vi "FillianVI.vi"() -> ()   [LabVIEW 2015]
uses:
  <vilib>/Utility/error.llb/Error Cluster From Error Code.vi
  <vilib>/ErrorRing/Error Ring.xnode
panel:
  out "Minimum voltage":dbl
  out "Max voltage":dbl
  out "Maximum temp":dbl
  out "Minimum temp":dbl
  out "Mean Temperature":dbl
  out "Mean voltage":dbl
  out "Warnings":errorcluster
  out "temp bat timeout":bool
  out "volt bat timeout":bool
  out "volt link timeout":bool
  out "temp link timeout":bool
  out "Link Quality 2":sgl
  out "Battery Voltage 2":sgl
  out "Battery Voltage":sgl
  out "Link Quality":sgl
  out "Voltage":sgl(graph)
  in  "stop":bool
  out "Temperature":sgl(graph)
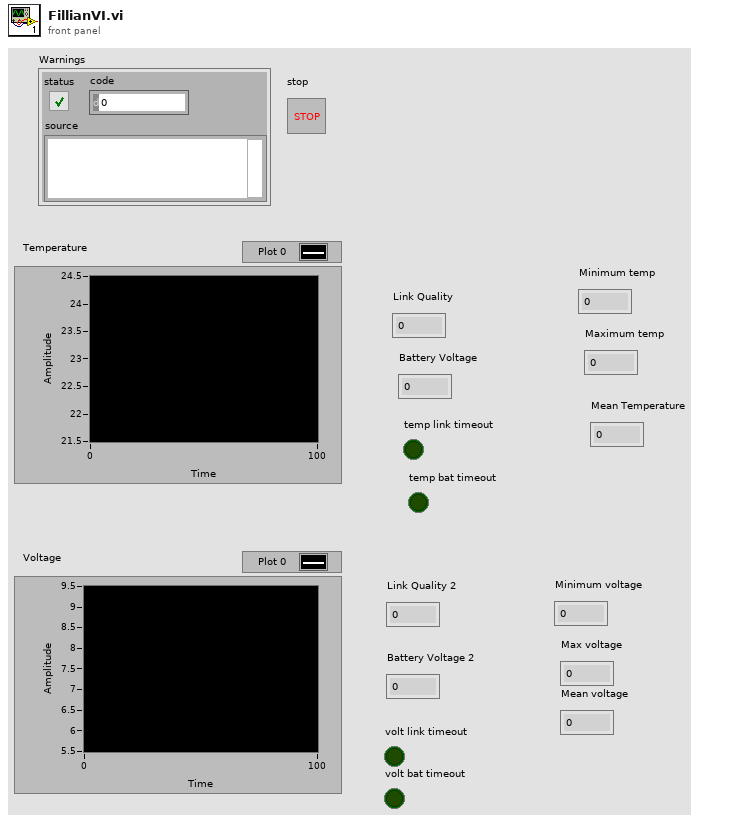
[diagram p1: front panel]
types:
  T1 = enum16{"open", "replace", "create", "open or create", "replace or create", "replace or create with confirmation"}
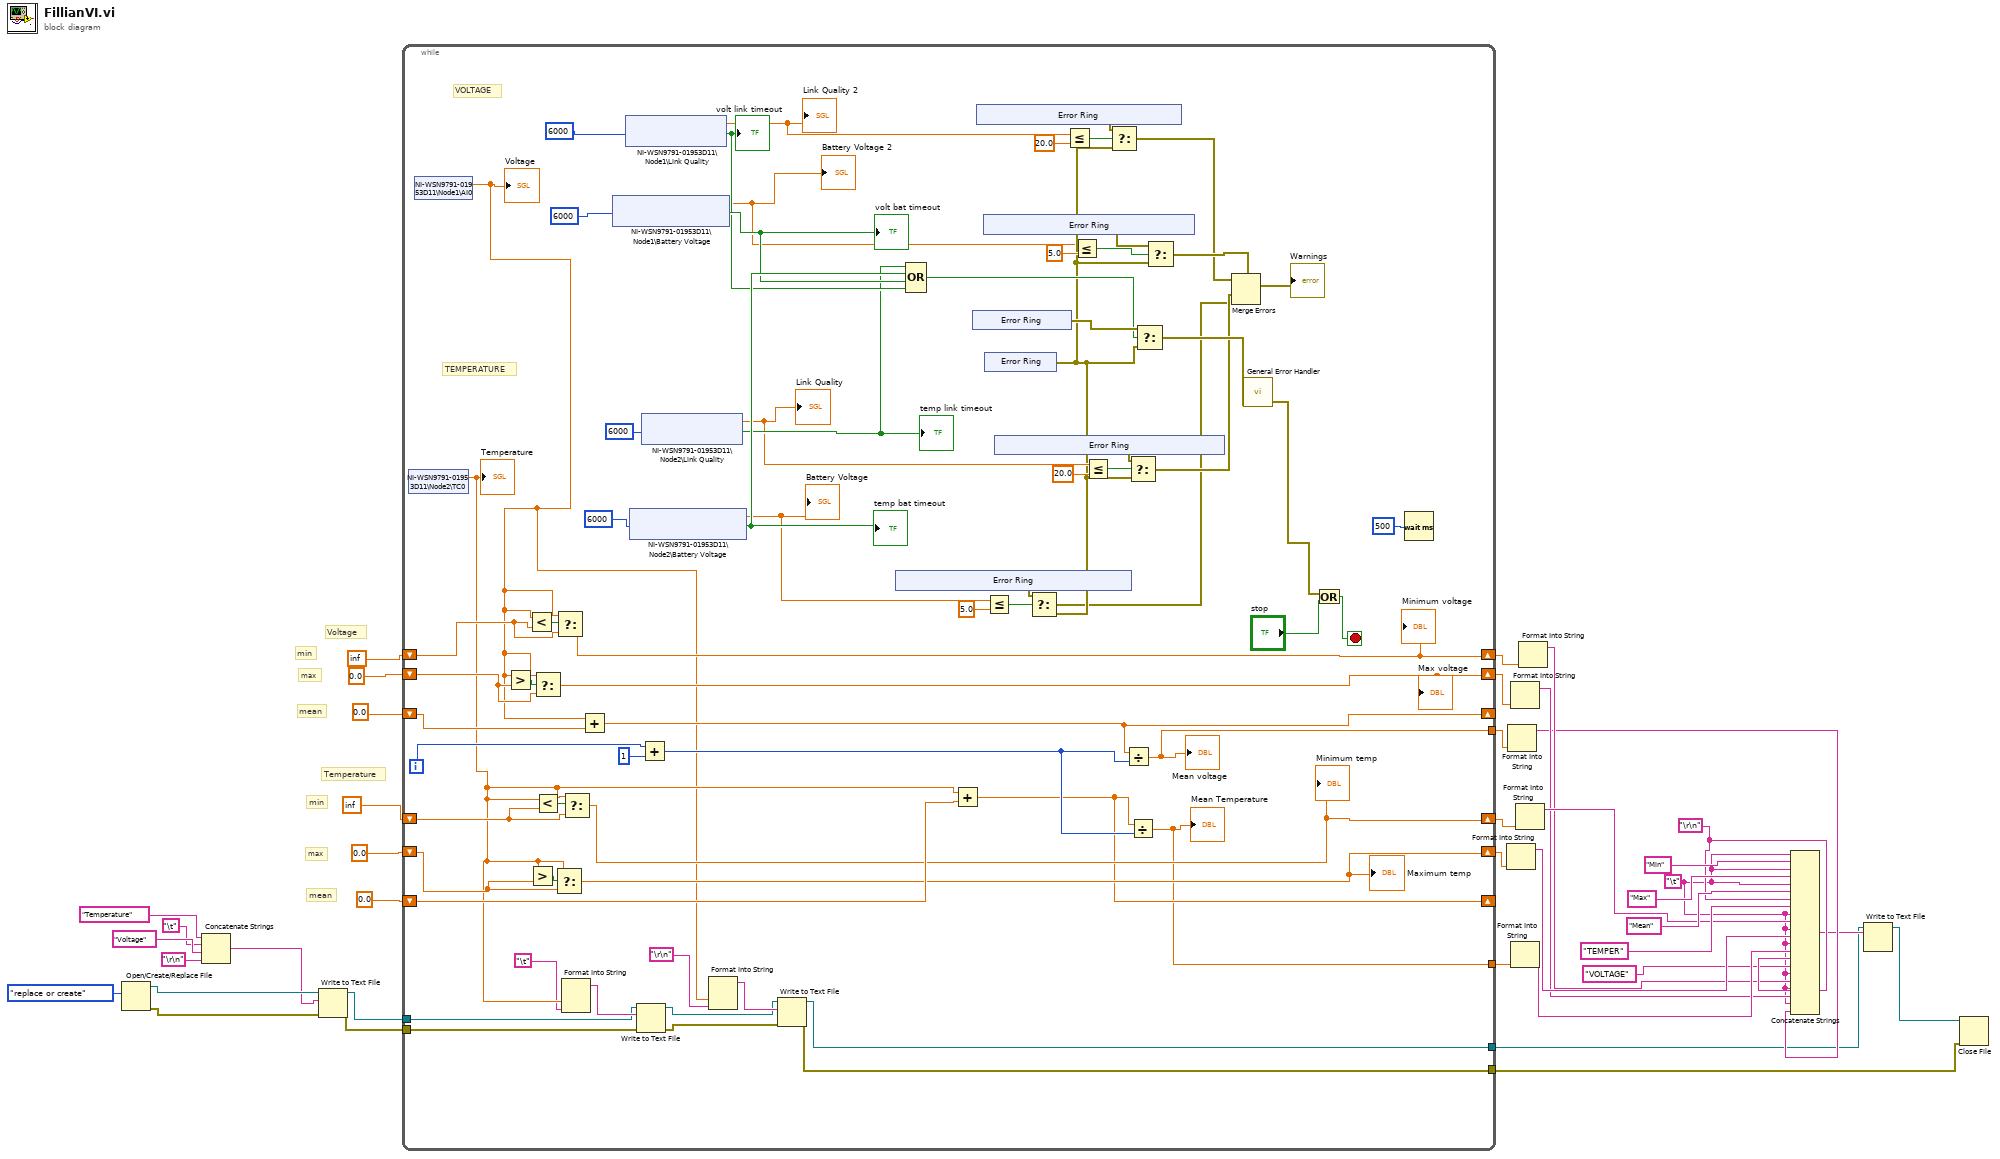
[diagram p0: block diagram]
diagram:
  w14 = "\r\n"
  w8 = "\t"
  # "max"
  # "mean"
  # "min"
  # "max"
  # "mean"
  # "min"
  # "Voltage"
  # "Temperature"
  n1 = Open/Create/Replace File(operation (0:open)=T1."replace or create") -> (refnum out=w32:refnum<file>, error out=w31:errorcluster)  [unwired: 5 in, 1 out]
  n2 = Concatenate Strings("Temperature" ("text"), "\t", "Voltage" ("text"), "\r\n") -> (w27:string)
  n3 = Write to Text File(file (use dialog)=w32, text=w27, error in=w31) -> (refnum out=w30:refnum<file>, error out=w29:errorcluster)  [unwired: 1 in, 1 out]
  n4 = while {
    shift-right: [w69] -> w11
    shift-left: inf -> [w70]
    shift-right: [w72] -> w12
    shift-left: 0.0 -> [w67]
    shift-right: [w55] -> w19
    shift-left: inf -> [w58]
    shift-right: [w56] -> w17
    shift-left: 0.0 -> [w57]
    shift-right: [w65] -> _
    shift-left: 0.0 -> [w68]
    shift-right: [w54] -> _
    shift-left: 0.0 -> [w59]
    tunnel: w30 -> [w49]
    tunnel: [w47] -> w5
    tunnel: w29 -> [w46]
    tunnel: [w44] -> w3
    tunnel: [w41] -> w2
    tunnel: [w40] -> w1
    i -> [w64]
    stop <- w98 stop-if-true
    # "VOLTAGE"
    # "TEMPERATURE"
    n5 = shared-variable "NI-WSN9791-01953D11\\Node2\\TC0"() -> (w51:sgl)  [unwired: 1 in, 1 out]
    "Temperature" <- w51
    n6 = shared-variable "NI-WSN9791-01953D11\\Node1\\AI0"() -> (w50:sgl)  [unwired: 1 in, 1 out]
    "Voltage" <- w50
    n7 = Greater?(x=w50, y=w67) -> (0:w73:bool)
    n8 = Less?(x=w50, y=w70) -> (x < y?=w71:bool)
    n9 = Greater?(x=w51, y=w57) -> (0:w61:bool)
    n10 = Select(t=w50, s=w73, f=w67) -> (s? t:f=w72:dbl)
    "Max voltage" <- w72
    n11 = Less?(x=w51, y=w58) -> (x < y?=w62:bool)
    n12 = Select(t=w51, s=w61, f=w57) -> (s? t:f=w56:dbl)
    "Maximum temp" <- w56
    n13 = Select(t=w50, s=w71, f=w70) -> (s? t:f=w69:dbl)
    "Minimum voltage" <- w69
    n14 = Format Into String(w51, "\t") -> (resulting string=w53:string)  [unwired: 3 in, 1 out]
    n15 = Select(t=w51, s=w62, f=w58) -> (s? t:f=w55:dbl)
    "Minimum temp" <- w55
    n16 = Add(x=w50, y=w68) -> (x+y=w65:dbl)
    n17 = shared-variable "NI-WSN9791-01953D11\\Node1\\Battery Voltage"(6000 ("ms timeout (0)")) -> (w66:sgl, w103:bool)  [unwired: 1 in, 1 out]
    "Battery Voltage 2" <- w66
    "volt bat timeout" <- w103
    n18 = shared-variable "NI-WSN9791-01953D11\\Node1\\Link Quality"(6000 ("ms timeout (0)")) -> (w87:sgl, w102:bool)  [unwired: 1 in, 1 out]
    "Link Quality 2" <- w87
    "volt link timeout" <- w102
    n19 = shared-variable "NI-WSN9791-01953D11\\Node2\\Battery Voltage"(6000 ("ms timeout (0)")) -> (w76:sgl, w104:bool)  [unwired: 1 in, 1 out]
    "Battery Voltage" <- w76
    "temp bat timeout" <- w104
    n20 = Write to Text File(file (use dialog)=w49, text=w53, error in=w46) -> (refnum out=w48:refnum<file>, error out=w45:errorcluster)  [unwired: 1 in, 1 out]
    n21 = Add(x=w64, y=1) -> (x+y=w60:i32)
    n22 = shared-variable "NI-WSN9791-01953D11\\Node2\\Link Quality"(6000 ("ms timeout (0)")) -> (w94:sgl, w95:bool)  [unwired: 1 in, 1 out]
    "Link Quality" <- w94
    "temp link timeout" <- w95
    n23 = Format Into String(w50, "\r\n") -> (resulting string=w52:string)  [unwired: 3 in, 1 out]
    n24 = Write to Text File(file (use dialog)=w48, text=w52, error in=w45) -> (refnum out=w47:refnum<file>, error out=w44:errorcluster)  [unwired: 1 in, 1 out]
    n25 = xnode "Error Ring"() -> ("error out"=w77:errorcluster)
    n26 = Compound Arithmetic op=OR(w95, w104, w103, w102) -> (w99:bool)
    n27 = Add(x=w51, y=w59) -> (x+y=w54:dbl)
    n28 = xnode "Error Ring"() -> ("error out"=w101:errorcluster)
    n29 = xnode "Error Ring"() -> ("error out"=w88:errorcluster)
    n30 = xnode "Error Ring"() -> ("error out"=w84:errorcluster)
    n31 = xnode "Error Ring"() -> ("error out"=w75:errorcluster)
    n32 = Less Or Equal?(x=w76, y=sgl 5.0) -> (x <= y?=w78:bool)
    n33 = xnode "Error Ring"() -> ("error out"=w91:errorcluster)
    n34 = Select(t=w77, s=w78, f=w75) -> (s? t:f=w74:errorcluster)
    n35 = Less Or Equal?(x=w87, y=sgl 20.0) -> (x <= y?=w89:bool)
    n36 = Less Or Equal?(x=w66, y=sgl 5.0) -> (x <= y?=w85:bool)
    n37 = Less Or Equal?(x=w94, y=sgl 20.0) -> (x <= y?=w92:bool)
    n38 = Select(t=w88, s=w89, f=w75) -> (s? t:f=w82:errorcluster)
    n39 = Divide(x=w65, y=w60) -> (x/y=w40:dbl)
    "Mean voltage" <- w40
    n40 = Select(t=w91, s=w92, f=w75) -> (s? t:f=w80:errorcluster)
    n41 = Divide(x=w54, y=w60) -> (x/y=w41:dbl)
    "Mean Temperature" <- w41
    n42 = Select(t=w101, s=w99, f=w75) -> (s? t:f=w100:errorcluster)
    n43 = Select(t=w84, s=w85, f=w75) -> (s? t:f=w83:errorcluster)
    n44 = Merge Errors(w82, w83, w80, w74) -> (→"Warnings":errorcluster)
    n45 = call <vilib>:"General Error Handler.vi"("error in (no error)"=w100) -> ("error out"=w96:errorcluster)  [unwired: 10 in, 4 out]
    n46 = Or(x=w96, y="stop") -> (x .or. y?=w98:bool)
    n47 = Wait (ms)(milliseconds to wait=u32 500) -> ()  [unwired: 1 out]
  }
  n48 = Format Into String(w17) -> (resulting string=w16:string)  [unwired: 3 in, 1 out]
  n49 = Format Into String(w1) -> (resulting string=w7:string)  [unwired: 3 in, 1 out]
  n50 = Format Into String(w12) -> (resulting string=w9:string)  [unwired: 3 in, 1 out]
  n51 = Format Into String(w2) -> (resulting string=w15:string)  [unwired: 3 in, 1 out]
  n52 = Format Into String(w19) -> (resulting string=w18:string)  [unwired: 3 in, 1 out]
  n53 = Format Into String(w11) -> (resulting string=w10:string)  [unwired: 3 in, 1 out]
  n54 = Concatenate Strings(w8, "Min", w8, "Max", w8, "Mean", w14, "TEMPER", w8, w18, w8, w16, w8, w15, w14, "VOLTAGE", w8, w10, w8, w9, w8, w7) -> (w6:string)
  n55 = Write to Text File(file (use dialog)=w5, text=w6) -> (refnum out=w4:refnum<file>)  [unwired: 2 in, 2 out]
  n56 = Close File(refnum=w4, error in=w3) -> ()  [unwired: 2 out]
